vi "Append Charact Result.vi"(0 "Path cal resut in":variant, 11 "error in (no error)":errorcluster) -> (15 "error out":errorcluster)   [LabVIEW 2023, in "RFFixtureCharact.Public.lvlib"]
uses:
  RFFixtureCharact.Public.lvlib
  Type Definitions/Collection Operation.ctl
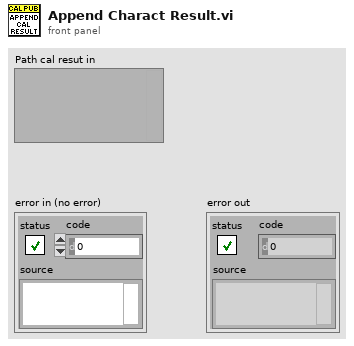
[diagram p1: front panel]
types:
  T1 = typedef "RFFixtureCharact.Public.lvlib/Collection Operation.ctl" = enum16{"Append", "Get", "Get All", "Clear"}
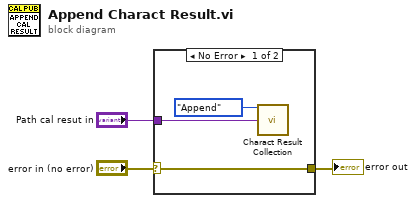
[diagram p0: block diagram]
diagram:
  n1 = case shown="No Error" "error in (no error)" {
    selector: "error in (no error)" -> [w4 w7]
    tunnel: "Path cal resut in" -> [w6 _]
    tunnel: [w4 w7] -> w1
    frame No Error {
      n2 = call "Charact Result Collection.vi"("Operation"=Collection_Operation."Append", "Path cal resut In"=w6) -> ()  [unwired: 12 in, 2 out]
    }
    frame Error {
    }
  }
  "error out" <- w1
